vi "Program04.vi"() -> ()   [LabVIEW 2020]
panel:
  out "SR1":i32
  out "Wynik":i32
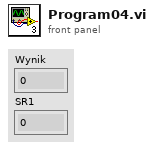
[diagram p1: front panel]
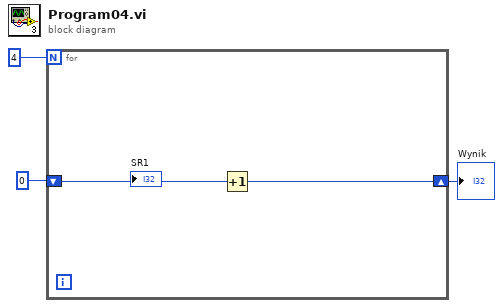
[diagram p0: block diagram]
diagram:
  n1 = for {
    N: 4 -> [_]
    shift-right: [w5] -> w1
    shift-left: 0 -> [w4]
    n2 = Increment(x=w4) -> (x+1=w5:i32)
    "SR1" <- w4
  }
  "Wynik" <- w1
